vi "Pusher_ClientExample_RT.vi"() -> ()   [LabVIEW 2009]
doc: "Run this VI on RT targets (such as cRIO etc)s"
uses:
  Client.lvclass
panel:
  in  "api_key":string
  in  "Channel":string="LvChannel"
  out "#PingPong":i32
  out "Data":string
  in  "stop":bool
  # "Instructions:\n1- Fill in your pusher API key\n2- Run the VI\n3- Use \"Event Creator\" tab on pusher.com to send events \nto your channel in the following format\n\nChannel Name: LvChannel\nEvent name: message\nEvent data: {\"name\":\"joe\",\"age\":\"30\"}"
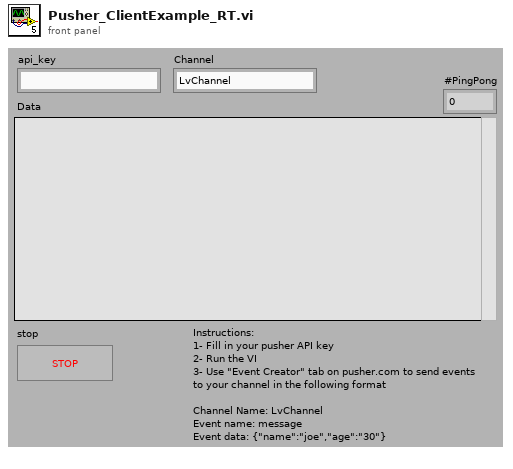
[diagram p1: front panel]
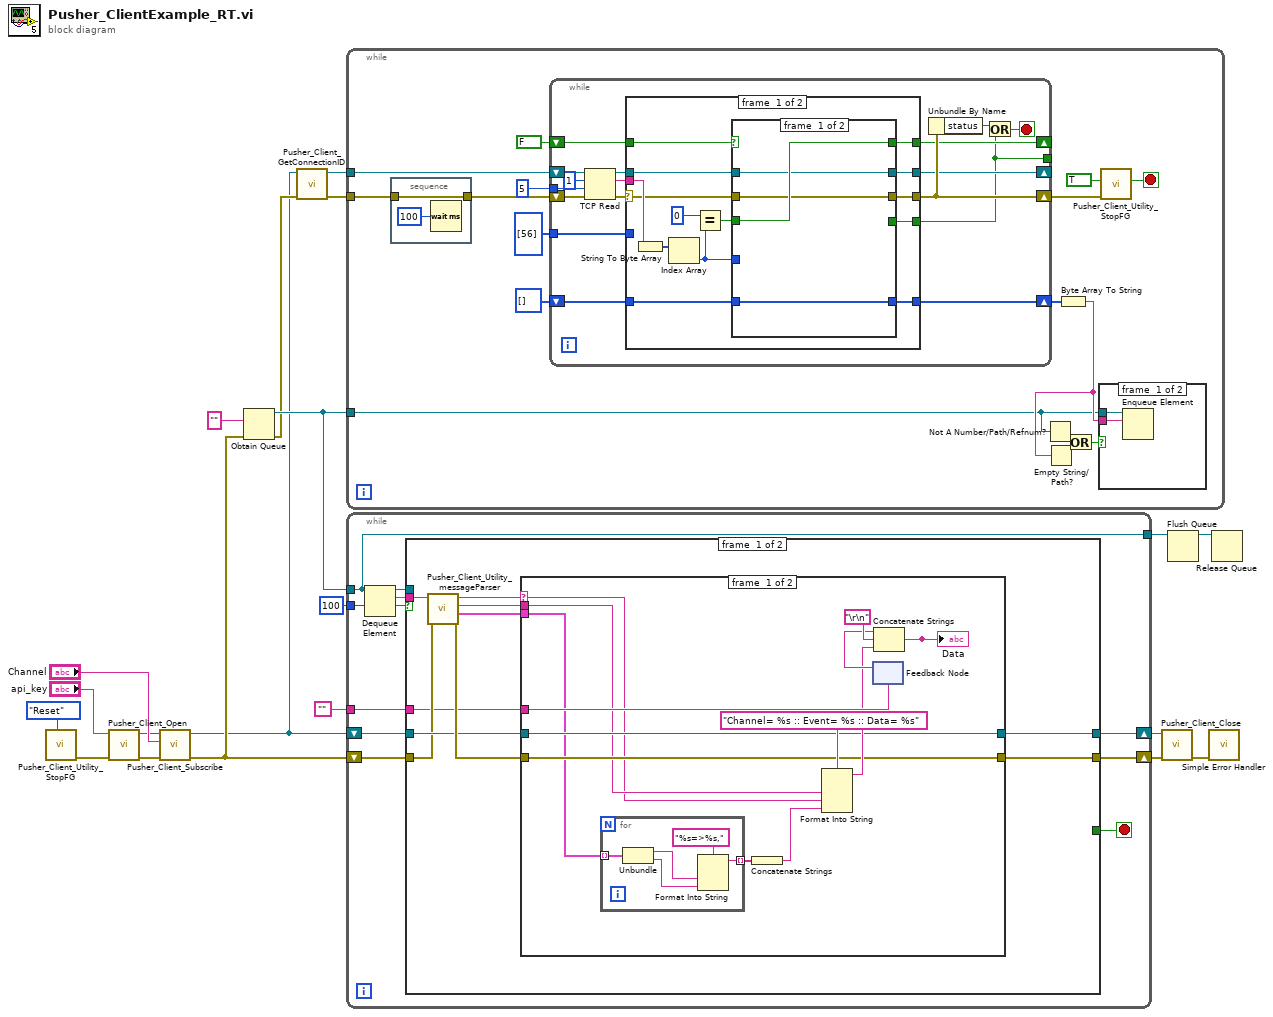
[diagram p0: block diagram]
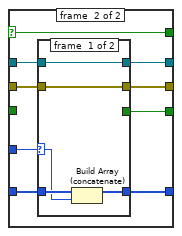
[diagram p3: hidden frame]
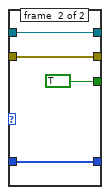
[diagram p4: hidden frame]
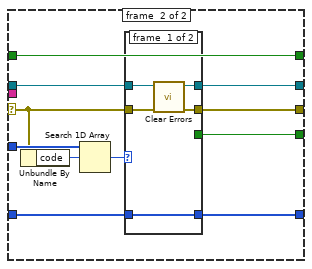
[diagram p5: hidden frame]
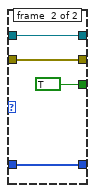
[diagram p6: hidden frame]
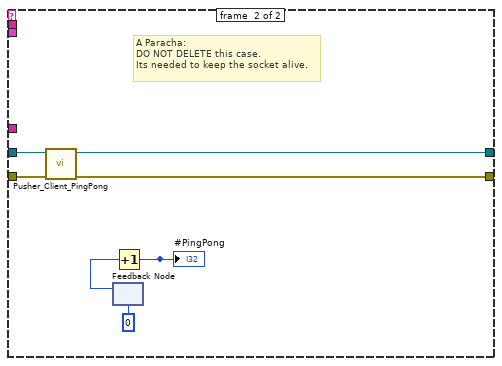
[diagram p7: hidden frame]
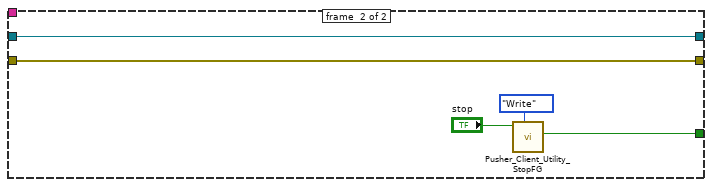
[diagram p8: hidden frame]
diagram:
  n1 = call "Pusher_Client_Utility_StopFG.vi"("Command"=enum16{"Write", "Read", "Reset"}."Reset") -> ("error out"=w14:errorcluster)  [unwired: 8 in, 2 out]
  n2 = call "Pusher_Client_Open.vi"("ErrIn"=w14, "api_key"="api_key") -> ("ErrOut"=w12:errorcluster, "Client out"=w11:refnum<class "Client.lvclass">)  [unwired: 8 in]
  n3 = call "Pusher_Client_Subscribe.vi"("ErrIn"=w12, "ChannelName"="Channel", "Client in"=w11) -> ("ErrOut"=w5:errorcluster, "Client out"=w3:refnum<class "Client.lvclass">)  [unwired: 7 in]
  n4 = Obtain Queue(element data type="", error in (no error)=w5) -> (queue out=w9:refnum<queue>, error out=w4:errorcluster)  [unwired: 3 in, 1 out]
  n5 = call "Pusher_Client_GetConnectionID.vi"("error in (no error)"=w4, "Client in"=w3) -> ("error out"=w1:errorcluster, "connectionID"=w2:refnum<k5>)  [unwired: 8 in]
  n6 = while {
    tunnel: w9 -> [w27]
    tunnel: w2 -> [w23]
    tunnel: w1 -> [w22]
    stop <- w24 stop-if-true
    n7 = stacked-sequence {
      tunnel: [w38] -> w21
      tunnel: w22 -> [w38]
      frame #0 {
        n8 = Wait (ms)(milliseconds to wait=u32 100) -> ()  [unwired: 1 out]
      }
    }
    n9 = while {
      tunnel: 5 -> [w54]
      tunnel: i32[] [56] -> [w51]
      shift-right: [w50] -> w26
      shift-left: w21 -> [w56]
      shift-right: [w49] -> _
      shift-left: w23 -> [w57]
      shift-right: [w46] -> w32
      shift-left: u8[] [] -> [w47]
      shift-right: [w42] -> _
      shift-left: FALSE -> [w43]
      tunnel: [w41] -> _
      stop <- w45 stop-if-true
      n10 = TCP Read(connection ID=w57, bytes to read=1, error in (no error)=w56, 9:w54) -> (connection ID out=w52:refnum<k5>, data out=w48:string, error out=w53:errorcluster)  [unwired: 1 in]
      n11 = case shown="No Error" w53 {
        selector: w53 -> [w65 w101]
        tunnel: w52 -> [w67 w99]
        tunnel: w51 -> [_ w103]
        tunnel: [w64 w100] -> w50
        tunnel: [w66 w98] -> w49
        tunnel: w48 -> [w70 _]
        tunnel: w47 -> [w69 w97]
        tunnel: [w68 w96] -> w46
        tunnel: [w63 w94] -> w41
        tunnel: [w59 w95] -> w42
        tunnel: w43 -> [w60 w95]
        frame #0 {
          n12 = String To Byte Array(string=w70) -> (unsigned byte array=w71:u8[])
          n13 = Index Array(array=w71) -> (element=w62:u8)  [unwired: 1 in]
          n14 = Equal?(x=u8 0, y=w62) -> (x = y?=w58:bool)
          n15 = case shown="True" w60 {
            selector: w60 -> [_ w76]
            tunnel: w62 -> [_ w84]
            tunnel: w69 -> [w72 w83]
            tunnel: [w72 w82] -> w68
            tunnel: w67 -> [w74 w81]
            tunnel: [w74 w80] -> w66
            tunnel: w65 -> [w73 w79]
            tunnel: [w73 w78] -> w64
            tunnel: [_ w77] -> w63
            tunnel: [w75 w76] -> w59
            tunnel: w58 -> [w75 _]
            frame #0 {
            }
            frame #1 {
              n16 = case shown="255" w84 {
                selector: w84 -> [w85 _]
                tunnel: w83 -> [w87 w93]
                tunnel: [w86 w93] -> w82
                tunnel: [w89 w92] -> w80
                tunnel: w81 -> [w89 w92]
                tunnel: [w88 w91] -> w78
                tunnel: w79 -> [w88 w91]
                tunnel: [_ TRUE] -> w77
                frame #0 {
                  n17 = Build Array (concatenate)(w87, w85) -> (w86:u8[])
                }
                frame #1 {
                }
              }
            }
          }
        }
        frame #1 {
          n18 = Unbundle By Name(w101) -> ("code"=w104:i32)
          n19 = Search 1D Array(1D array=w103, element=w104) -> (index of element=w102:i32)  [unwired: 1 in]
          n20 = case shown="0, Default" w102 {
            tunnel: w101 -> [w108 w112]
            tunnel: [w107 w112] -> w100
            tunnel: [w106 w111] -> w98
            tunnel: w99 -> [w106 w111]
            tunnel: [w105 w110] -> w96
            tunnel: w97 -> [w105 w110]
            tunnel: [_ TRUE] -> w94
            frame #0 {
              n21 = call <vilib>:"Clear Errors.vi"("error in (no error)"=w108) -> ("error out"=w107:errorcluster)  [unwired: 6 in]
            }
            frame #1 {
            }
          }
        }
      }
      n22 = Unbundle By Name(w50) -> ("status"=w44:bool)
      n23 = Or(x=w44, y=w41) -> (x .or. y?=w45:bool)
    }
    n24 = Not A Number/Path/Refnum?(number/path/refnum=w27) -> (NaN/Path/Refnum?=w31:bool)
    n25 = Byte Array To String(unsigned byte array=w32) -> (string=w28:string)
    n26 = Empty String/Path?(string/path=w28) -> (empty?=w30:bool)
    n27 = Or(x=w31, y=w30) -> (x .or. y?=w29:bool)
    n28 = case shown="False" w29 {
      tunnel: w28 -> [w39 _]
      tunnel: w27 -> [w40 _]
      frame #0 {
        n29 = Enqueue Element(queue=w40, element=w39) -> ()  [unwired: 2 in, 3 out]
      }
      frame #1 {
      }
    }
    n30 = call "Pusher_Client_Utility_StopFG.vi"("error in (no error)"=w26, "Stop on Error?"=TRUE) -> ("Latched Stop"=w24:bool)  [unwired: 7 in, 2 out]
  }
  n31 = while {
    shift-right: [w120] -> w16
    shift-left: w5 -> [w121]
    shift-right: [w119] -> w17
    shift-left: w3 -> [w122]
    tunnel: "" -> [w118]
    tunnel: w9 -> [w113]
    tunnel: 100 -> [w117]
    tunnel: [w113] -> w7
    stop <- w123 stop-if-true
    n32 = Dequeue Element(queue=w113, timeout in ms (-1)=w117) -> (queue out=w115:refnum<queue>, element=w114:string, timed out?=w116:bool)  [unwired: 1 in, 1 out]
    n33 = case shown="False" w116 {
      tunnel: [_ w160] -> w123
      tunnel: w122 -> [w129 w163]
      tunnel: w121 -> [w128 w159]
      tunnel: [w126 w159] -> w120
      tunnel: [w127 w163] -> w119
      tunnel: w118 -> [w125 _]
      tunnel: w115 -> [_ _]
      tunnel: w114 -> [w130 _]
      frame #0 {
        n34 = call "Pusher_Client_Utility_messageParser.vi"("ErrIn"=w128, "message"=w130) -> ("ErrOut"=w132:errorcluster, "data"=w131:cluster{"name":string, "value":string}[], "Channel"=w124:string, "Event"=w133:string)  [unwired: 5 in, 1 out]
        n35 = case shown="\"False\", Default" w133 {
          selector: w133 -> [w134 _]
          tunnel: w125 -> [w145 _]
          tunnel: w132 -> [w140 w158]
          tunnel: w129 -> [w139 w157]
          tunnel: [w139 w156] -> w127
          tunnel: [w140 w155] -> w126
          tunnel: w124 -> [w135 _]
          tunnel: w131 -> [w138 _]
          frame #0 {
            n36 = for {
              tunnel: w138 -> [w151] mode=indexing
              tunnel: [w147] -> w137 mode=indexing
              n37 = Unbundle(w151) -> ("name"=w149:string, "value"=w148:string)
              n38 = Format Into String(format string="%s=>%s,", w149, w148) -> (resulting string=w147:string)  [unwired: 2 in, 1 out]
            }
            n39 = Concatenate Strings(w137) -> (w136:string)
            n40 = Format Into String(format string="Channel= %s :: Event= %s :: Data= %s", w135, w134, w136) -> (resulting string=w141:string)  [unwired: 2 in, 1 out]
            n41 = feedback #1(w145) -> (w143:string)
            n42 = Concatenate Strings(w143, "\r\n", w141) -> (w144:string)
            "Data" <- w144
          }
          frame #1 {
            # "A Paracha:\nDO NOT DELETE this case.\nIts needed to keep the socket alive."
            n43 = call "Pusher_Client_PingPong.vi"("ErrIn"=w158, "Client in"=w157) -> ("ErrOut"=w155:errorcluster, "Client out"=w156:refnum<class "Client.lvclass">)  [unwired: 8 in]
            n44 = feedback #2(0) -> (w153:i32)
            n45 = Increment(x=w153) -> (x+1=w152:i32)
            "#PingPong" <- w152
          }
        }
      }
      frame #1 {
        n46 = call "Pusher_Client_Utility_StopFG.vi"("Command"=enum16{"Write", "Read", "Reset"}."Write", "Stop?"="stop") -> ("Latched Stop"=w160:bool)  [unwired: 7 in, 2 out]
      }
    }
  }
  n47 = call "Pusher_Client_Close.vi"("ErrIn"=w16, "Client in"=w17) -> ("ErrOut"=w19:errorcluster)  [unwired: 9 in]
  n48 = Flush Queue(queue=w7) -> (queue out=w6:refnum<queue>)  [unwired: 1 in, 2 out]
  n49 = call <vilib>:"Simple Error Handler.vi"("error in (no error)"=w19) -> ()  [unwired: 4 in, 5 out]
  n50 = Release Queue(queue=w6) -> ()  [unwired: 2 in, 3 out]
